vi "LaunchBrain.vi"   [LabVIEW 2011]
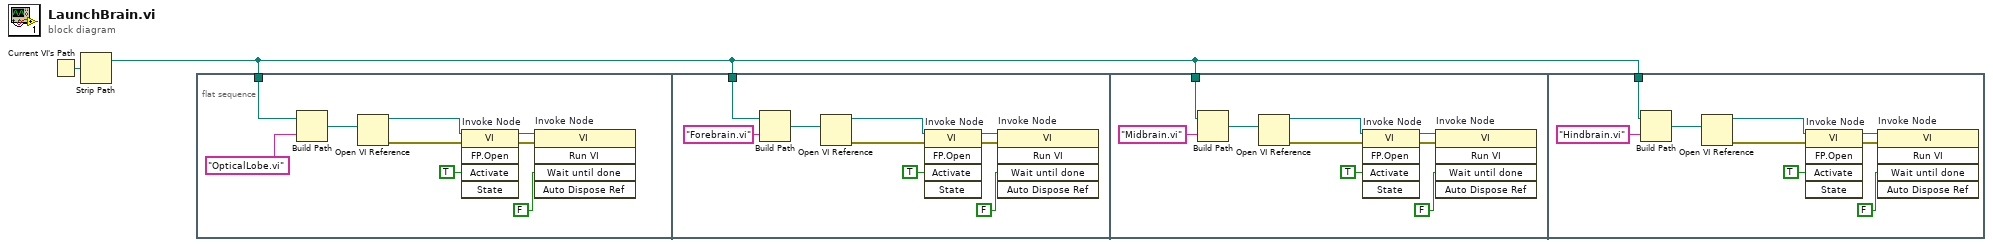
[diagram p0: block diagram]
diagram:
  n1 = Current VI's Path() -> (path=w2:path)
  n2 = Strip Path(path=w2) -> (stripped path=w1:path)  [unwired: 1 out]
  n3 = flat-sequence {
    tunnel: w1 -> [w3]
    tunnel: w1 -> [w12]
    tunnel: w1 -> [w24]
    tunnel: w1 -> [w33]
    frame #0 {
      n4 = Build Path(base path=w3, name or relative path="OpticalLobe.vi") -> (appended path=w7:path)
      n5 = Open VI Reference(vi path=w7) -> (vi reference=w5:refnum<vi>, error out=w8:errorcluster)  [unwired: 5 in]
      n6 = invoke on="Invoke Node" class="VI" method="FP.Open"(reference=w5, error in=w8, "Activate"=TRUE ("Activate?")) -> (reference out=w10:refnum<vi>, error out=w4:errorcluster)  [unwired: 2 in, 3 out]
      n7 = invoke on="Invoke Node" class="VI" method="Run VI"(reference=w10, error in=w4, "Wait until done"=FALSE ("Wait Until Done")) -> ()  [unwired: 2 in, 5 out]
    }
    frame #1 {
      n8 = Build Path(base path=w12, name or relative path="Forebrain.vi") -> (appended path=w16:path)
      n9 = Open VI Reference(vi path=w16) -> (vi reference=w14:refnum<vi>, error out=w17:errorcluster)  [unwired: 5 in]
      n10 = invoke on="Invoke Node" class="VI" method="FP.Open"(reference=w14, error in=w17, "Activate"=TRUE ("Activate?")) -> (reference out=w19:refnum<vi>, error out=w13:errorcluster)  [unwired: 2 in, 3 out]
      n11 = invoke on="Invoke Node" class="VI" method="Run VI"(reference=w19, error in=w13, "Wait until done"=FALSE ("Wait Until Done")) -> ()  [unwired: 2 in, 5 out]
    }
    frame #2 {
      n12 = Build Path(base path=w24, name or relative path="Midbrain.vi") -> (appended path=w25:path)
      n13 = Open VI Reference(vi path=w25) -> (vi reference=w22:refnum<vi>, error out=w29:errorcluster)  [unwired: 5 in]
      n14 = invoke on="Invoke Node" class="VI" method="FP.Open"(reference=w22, error in=w29, "Activate"=TRUE ("Activate?")) -> (reference out=w27:refnum<vi>, error out=w21:errorcluster)  [unwired: 2 in, 3 out]
      n15 = invoke on="Invoke Node" class="VI" method="Run VI"(reference=w27, error in=w21, "Wait until done"=FALSE ("Wait Until Done")) -> ()  [unwired: 2 in, 5 out]
    }
    frame #3 {
      n16 = Build Path(base path=w33, name or relative path="Hindbrain.vi") -> (appended path=w34:path)
      n17 = Open VI Reference(vi path=w34) -> (vi reference=w31:refnum<vi>, error out=w38:errorcluster)  [unwired: 5 in]
      n18 = invoke on="Invoke Node" class="VI" method="FP.Open"(reference=w31, error in=w38, "Activate"=TRUE ("Activate?")) -> (reference out=w36:refnum<vi>, error out=w30:errorcluster)  [unwired: 2 in, 3 out]
      n19 = invoke on="Invoke Node" class="VI" method="Run VI"(reference=w36, error in=w30, "Wait until done"=FALSE ("Wait Until Done")) -> ()  [unwired: 2 in, 5 out]
    }
  }
